vi "Material-CheckifZero.vi"(0 "DBL liner in":dbl, 1 "Digital in":refnum<vi>) -> ()   [LabVIEW 2013, in "Material-RunTest.lvclass"]
uses:
  Material-RunTest.lvclass
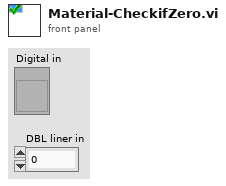
[diagram p1: front panel]
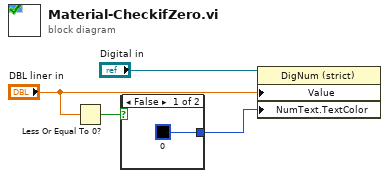
[diagram p0: block diagram]
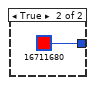
[diagram p2: hidden frame]
diagram:
  n1 = Less Or Equal To 0?(x="DBL liner in") -> (x <= 0?=w2:bool)
  n2 = case shown="False" w2 {
    tunnel: [u32 0 u32 16711680] -> w1
    frame False {
    }
    frame True {
    }
  }
  n3 = property on="Property Node" class="DigNum (strict)"(reference="Digital in", "Value"="DBL liner in", "NumText.TextColor"=w1) -> ()  [unwired: 1 in, 2 out]
